vi "pinout-settings.vi"(0 "main_light_pin":u8=8, 1 "main_fan_pin":u8=9, 2 "closed_roof_distance":dbl=3.0, 3 "roof_sensor_data_pin":u8=4, 4 "roof_sensor_echo_pin":u8=5, 5 "outdoor_temp_pin":u8=2, 6 "light_on_threshold":u8=30, 7 "indoor_light_sensor_pin":u8=4, 12 "LabVIEW Web Service Request":refnum<class "Web Request.lvclass">) -> ()   [LabVIEW 2023]
uses:
  PinoutSettings.vi
  <vilib>/Utility/config.llb/NI_LVConfig.lvlib
  <vilib>/Utility/config.llb/Write Key (U32).vi
  <vilib>/Utility/config.llb/Write Key (Double).vi
  <vilib>/wsapi/Web Request.lvclass
panel:
  in  "configuration file path":path=path "C:/Users/Toni/Desktop/pinout.ini"
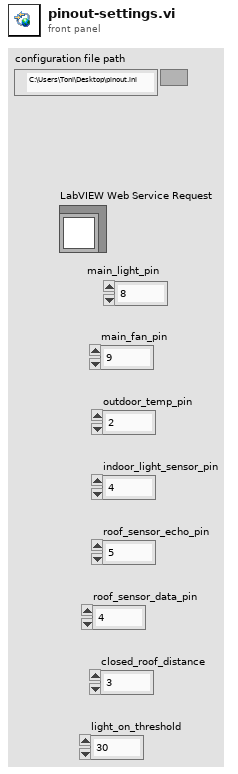
[diagram p1: front panel]
types:
  T1 = typedef "NI_LVConfig.lvlib/Config Data RefNum.ctl" = refnum<k1>
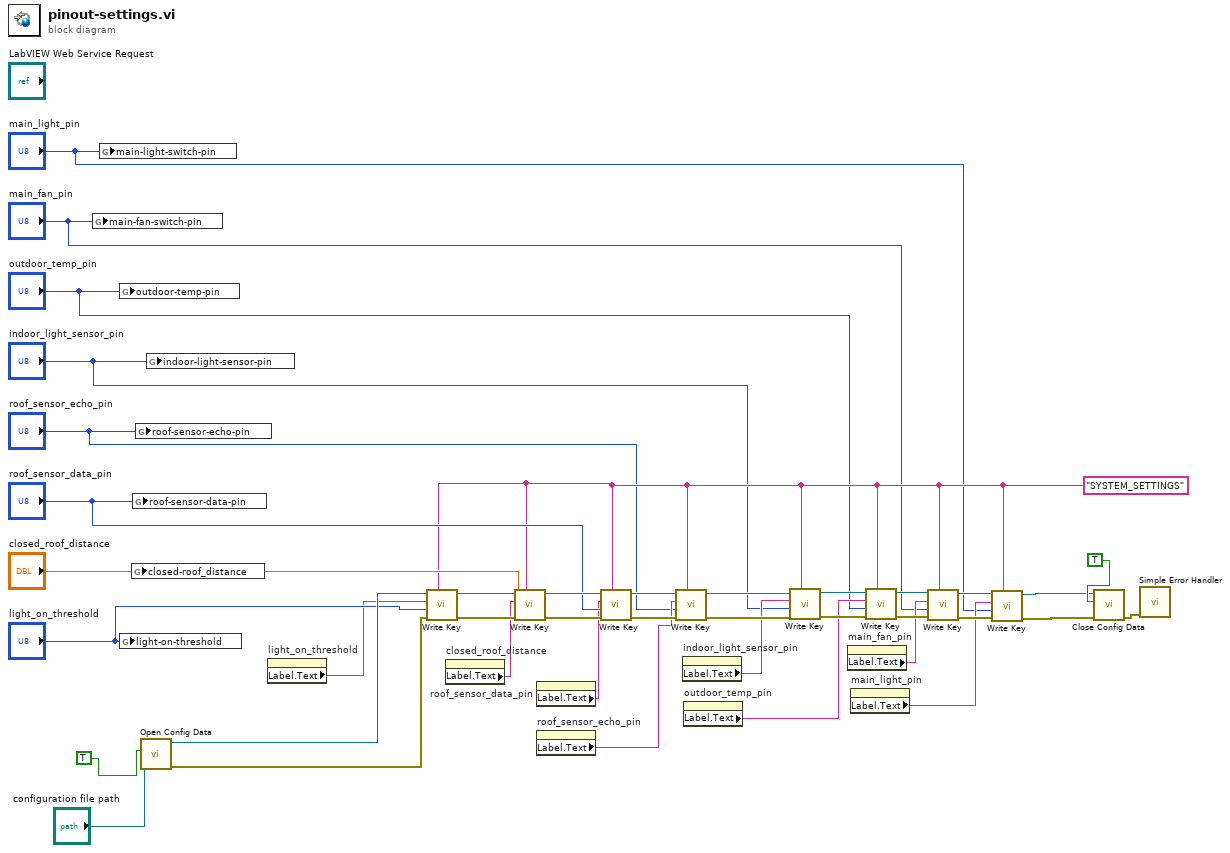
[diagram p0: block diagram]
diagram:
  w11 = "SYSTEM_SETTINGS" ("section")
  n1 = global write "PinoutSettings.vi" "main-fan-switch-pin"("main_fan_pin") -> ()
  n2 = global write "PinoutSettings.vi" "main-light-switch-pin"("main_light_pin") -> ()
  n3 = global write "PinoutSettings.vi" "outdoor-temp-pin"("outdoor_temp_pin") -> ()
  n4 = global write "PinoutSettings.vi" "light-on-threshold"("light_on_threshold") -> ()
  n5 = global write "PinoutSettings.vi" "closed-roof_distance"("closed_roof_distance") -> ()
  n6 = global write "PinoutSettings.vi" "roof-sensor-data-pin"("roof_sensor_data_pin") -> ()
  n7 = global write "PinoutSettings.vi" "roof-sensor-echo-pin"("roof_sensor_echo_pin") -> ()
  n8 = call <vilib>:"Open Config Data.vi"("create file if necessary (T)"=TRUE, "configuration file path"="configuration file path") -> ("error out"=w39:errorcluster, "refnum"=w34:T1)  [unwired: 7 in, 1 out]
  n9 = global write "PinoutSettings.vi" "indoor-light-sensor-pin"("indoor_light_sensor_pin") -> ()
  n10 = property on="light_on_threshold" class="DigNum (strict)"() -> ("Label.Text"=w32:string)  [unwired: 2 in, 2 out]
  n11 = call-poly <vilib>:"Write Key.vi"("section"=w11, "error in (no error)"=w39, "value"="light_on_threshold", "key"=w32, "refnum"=w34) -> ("error out"=w31:errorcluster, "refnum out"=w30:T1)  [unwired: 4 in, 1 out]
  n12 = property on="closed_roof_distance" class="DigNum (strict)"() -> ("Label.Text"=w28:string)  [unwired: 2 in, 2 out]
  n13 = call-poly <vilib>:"Write Key.vi"("section"=w11, "error in (no error)"=w31, "value"="closed_roof_distance", "key"=w28, "refnum"=w30) -> ("error out"=w27:errorcluster, "refnum out"=w26:T1)  [unwired: 4 in, 1 out]
  n14 = property on="roof_sensor_data_pin" class="DigNum (strict)"() -> ("Label.Text"=w24:string)  [unwired: 2 in, 2 out]
  n15 = property on="roof_sensor_echo_pin" class="DigNum (strict)"() -> ("Label.Text"=w10:string)  [unwired: 2 in, 2 out]
  n16 = call-poly <vilib>:"Write Key.vi"("section"=w11, "error in (no error)"=w27, "value"="roof_sensor_data_pin", "key"=w24, "refnum"=w26) -> ("error out"=w13:errorcluster, "refnum out"=w15:T1)  [unwired: 4 in, 1 out]
  n17 = call-poly <vilib>:"Write Key.vi"("section"=w11, "error in (no error)"=w13, "value"="roof_sensor_echo_pin", "key"=w10, "refnum"=w15) -> ("error out"=w19:errorcluster, "refnum out"=w20:T1)  [unwired: 4 in, 1 out]
  n18 = property on="indoor_light_sensor_pin" class="DigNum (strict)"() -> ("Label.Text"=w9:string)  [unwired: 2 in, 2 out]
  n19 = property on="outdoor_temp_pin" class="DigNum (strict)"() -> ("Label.Text"=w8:string)  [unwired: 2 in, 2 out]
  n20 = call-poly <vilib>:"Write Key.vi"("section"=w11, "error in (no error)"=w19, "value"="indoor_light_sensor_pin", "key"=w9, "refnum"=w20) -> ("error out"=w18:errorcluster, "refnum out"=w21:T1)  [unwired: 4 in, 1 out]
  n21 = property on="main_fan_pin" class="DigNum (strict)"() -> ("Label.Text"=w7:string)  [unwired: 2 in, 2 out]
  n22 = property on="main_light_pin" class="DigNum (strict)"() -> ("Label.Text"=w6:string)  [unwired: 2 in, 2 out]
  n23 = call-poly <vilib>:"Write Key.vi"("section"=w11, "error in (no error)"=w18, "value"="outdoor_temp_pin", "key"=w8, "refnum"=w21) -> ("error out"=w17:errorcluster, "refnum out"=w22:T1)  [unwired: 4 in, 1 out]
  n24 = call-poly <vilib>:"Write Key.vi"("section"=w11, "error in (no error)"=w17, "value"="main_fan_pin", "key"=w7, "refnum"=w22) -> ("error out"=w16:errorcluster, "refnum out"=w23:T1)  [unwired: 4 in, 1 out]
  n25 = call-poly <vilib>:"Write Key.vi"("section"=w11, "error in (no error)"=w16, "value"="main_light_pin", "key"=w6, "refnum"=w23) -> ("error out"=w12:errorcluster, "refnum out"=w14:T1)  [unwired: 4 in, 1 out]
  n26 = call <vilib>:"Close Config Data.vi"("error in (no error)"=w12, "write file if changed (T)"=TRUE, "refnum"=w14) -> ("error out"=w38:errorcluster)  [unwired: 7 in, 1 out]
  n27 = call <vilib>:"Simple Error Handler.vi"("error in (no error)"=w38) -> ()  [unwired: 4 in, 5 out]
